vi "AOMReadWrite.vi"(7 "Enum":enum16{"READ", "WRITE"}(ring), 8 "error in":errorcluster, 11 "XAOMsetting":T1(xcontrol)) -> (0 "error out":errorcluster, 2 "AOM signal":fxp<+/-,19,14>, 3 "Photodiode":dbl)   [LabVIEW 2019]
uses:
  controls/xAOMSettings/XAOMsetting.xctl
  <vilib>/Utility/error.llb/Error Cluster From Error Code.vi
  <vilib>/rvi/errors/niLvFpgaAdjustHostInterfaceError.vi
  <vilib>/rvi/interface/nirviReadWriteControl/nirviReadWriteControl.xnode
  <vilib>/rvi/interface/Simulation/niFpgaSimulationCallBeginRW.vi
  <vilib>/ptbypt/NI_PtbyPt.lvlib
  NiFpgaLv.dll
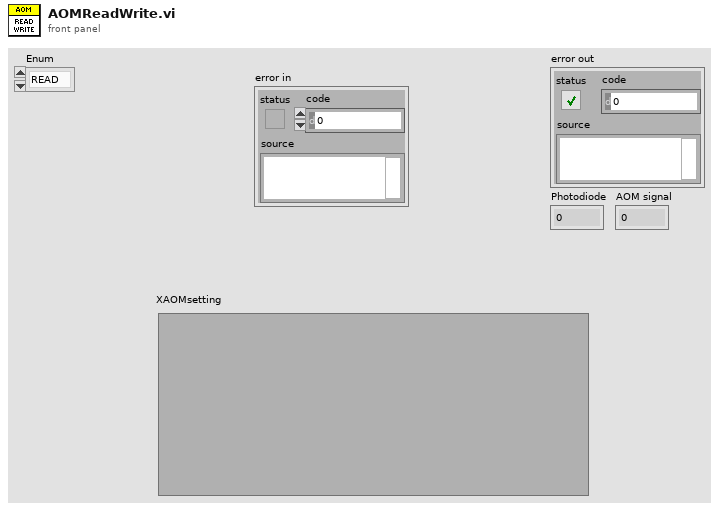
[diagram p1: front panel]
types:
  T1 = cluster{"HighPowerNum":dbl, "LowPowerNum":dbl, "PIDnum":dbl, "DeltaFreq":dbl, "BaseFreq":dbl, "AOMout":dbl, "ButtonSelected":enum16{"PID", "Low", "High"}, "AO3":bool}
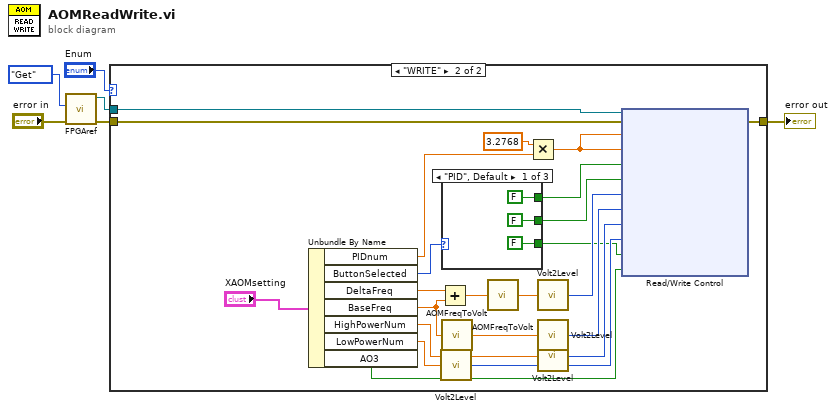
[diagram p0: block diagram]
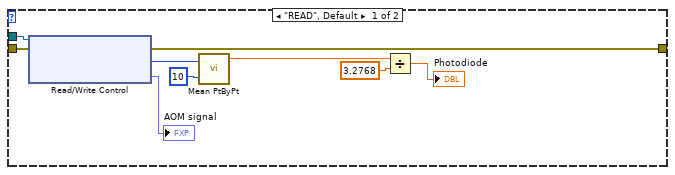
[diagram p2: hidden frame]
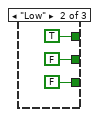
[diagram p3: hidden frame]
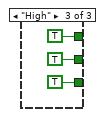
[diagram p4: hidden frame]
diagram:
  n1 = call "FPGAref.vi"("error in"="error in", "Enum"=enum16{"Set", "Get"}."Get") -> ("error out"=w3:errorcluster, "FPGA VI Reference Out 2"=w4:refnum<k20>)  [unwired: 4 in]
  n2 = case shown="\"WRITE\"" "Enum" {
    tunnel: w4 -> [w15 w35]
    tunnel: w3 -> [w14 w34]
    tunnel: [w9 w26] -> w1
    frame "READ", Default {
      n3 = xnode "Read/Write Control"("FPGA VI Reference In"=w15, "error in"=w14) -> ("error out"=w9:errorcluster, "Filtered Input"=w11:i16, "Control Signal / mV"=→"AOM signal":fxp<+/-,19,14>)  [unwired: 1 out]
      n4 = call <vilib>:"Mean PtByPt.vi"("x"=w11, "sample length"=10) -> ("mean"=w10:dbl)  [unwired: 2 in, 1 out]
      n5 = Divide(x=w10, y=3.2768) -> (x/y=→"Photodiode":dbl)
    }
    frame "WRITE" {
      n6 = Unbundle By Name("XAOMsetting") -> ("PIDnum"=w37:dbl, "ButtonSelected"=w24:enum16{"PID", "Low", "High"}, "DeltaFreq"=w28:dbl, "BaseFreq"=w27:dbl, "HighPowerNum"=w20:dbl, "LowPowerNum"=w21:dbl, "AO3"=w16:bool)
      n7 = Add(x=w28, y=w27) -> (x+y=w33:dbl)
      n8 = call "Volt2Level.vi"("voltage /V"=w21) -> ("level"=w18:i16)
      n9 = case shown="\"PID\", Default" w24 {
        tunnel: [FALSE TRUE TRUE] -> w23
        tunnel: [FALSE FALSE TRUE] -> w22
        tunnel: [FALSE FALSE TRUE] -> w17
        frame "PID", Default {
        }
        frame "Low" {
        }
        frame "High" {
        }
      }
      n10 = call "AOMFreqToVolt.vi"("AOM freq"=w27) -> ("AOM voltage"=w31:dbl)
      n11 = call "AOMFreqToVolt.vi"("AOM freq"=w33) -> ("AOM voltage"=w32:dbl)
      n12 = Multiply(x=3.2768, y=w37) -> (x*y=w36:dbl)
      n13 = call "Volt2Level.vi"("voltage /V"=w32) -> ("level"=w30:i16)
      n14 = call "Volt2Level.vi"("voltage /V"=w31) -> ("level"=w29:i16)
      n15 = call "Volt2Level.vi"("voltage /V"=w20) -> ("level"=w19:i16)
      n16 = xnode "Read/Write Control"("FPGA VI Reference In"=w35, "error in"=w34, "Setpoint (H)"=w36, "Setpoint (L)"=w36, "override noise eater?"=w23, "High power"=w22, "AO3 on"=w30, "AO3 off"=w29, "AO4 on"=w19, "AO4 off"=w18, "AO4"=w17, "AO3"=w16) -> ("error out"=w26:errorcluster)  [unwired: 1 out]
    }
  }
  "error out" <- w1
